vi "Duration to String.vi"(11 "Duration (s)":dbl) -> (3 "Duration String":string)   [LabVIEW 2019, in "Muon Data Post-Processing.lvlib"]
uses:
  Muon Data Post-Processing.lvlib
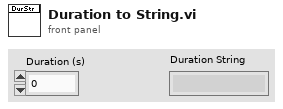
[diagram p1: front panel]
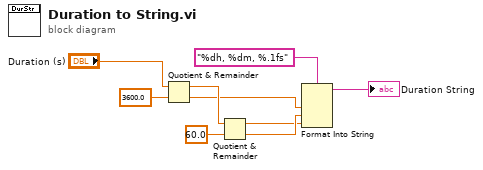
[diagram p0: block diagram]
diagram:
  n1 = Quotient & Remainder(x="Duration (s)", y=3600.0) -> (x-y*floor(x/y)=w7:dbl, floor(x/y)=w5:dbl)
  n2 = Quotient & Remainder(x=w7, y=60.0) -> (x-y*floor(x/y)=w3:dbl, floor(x/y)=w4:dbl)
  n3 = Format Into String(format string="%dh, %dm, %.1fs", w5, w4, w3) -> (resulting string=→"Duration String":string)  [unwired: 2 in, 1 out]
